vi "GEMM(LabVIEW).vi"() -> ()   [LabVIEW 2020]
uses:
  4e24d26d-fcbb-44a5-9aa8-75639d06e416.vi
  <vilib>/Analysis/baseanly.llb/Real A x B.vi
  2ed5783d-9886-4979-abaf-b24675aa47c9.vi
  <vilib>/Analysis/baseanly.llb/Mean (DBL).vi
  <vilib>/Utility/High Resolution Relative Seconds.vi
  <vilib>/Utility/file.llb/Write Delimited Spreadsheet (string).vi
  <vilib>/Analysis/NI_AALBase.lvlib
panel:
  in  "Benchmark Params":cluster{"Size":i32, "Iteration":i32}[](array[cluster])=[{"Size"=64, "Iteration"=20}, {"Size"=128, "Iteration"=20}, {"Size"=256, "Iteration"=20}, {"Size"=512, "Iteration"=20}, {"Size"=1024, "Iteration"=20}, {"Size"=2048, "Iteration"=20}, {"Size"=4096, "Iteration"=20}, {"Size"=8192, "Iteration"=3}]
  out "Results(ms)":dbl[](array[numeric])=[0.01173999989987351, 0.11100666645991926, 0.5743133331028124, 4.497079999176397, 36.276073333040884, 300.8564533326232, 2447.210946666261, 19172.94122000094] format="%.6f"
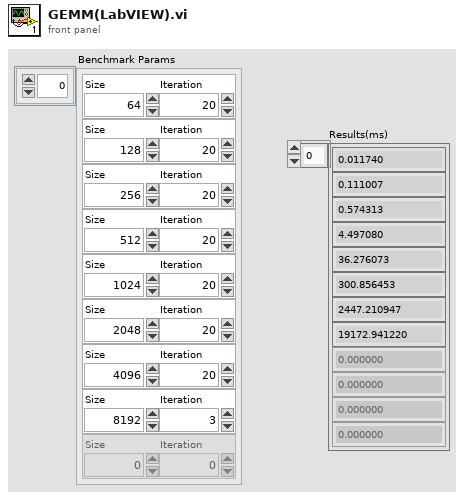
[diagram p1: front panel]
types:
  T1 = typedef "NI_Matrix.lvlib/RealMatrix.ctl" = dbl[][]
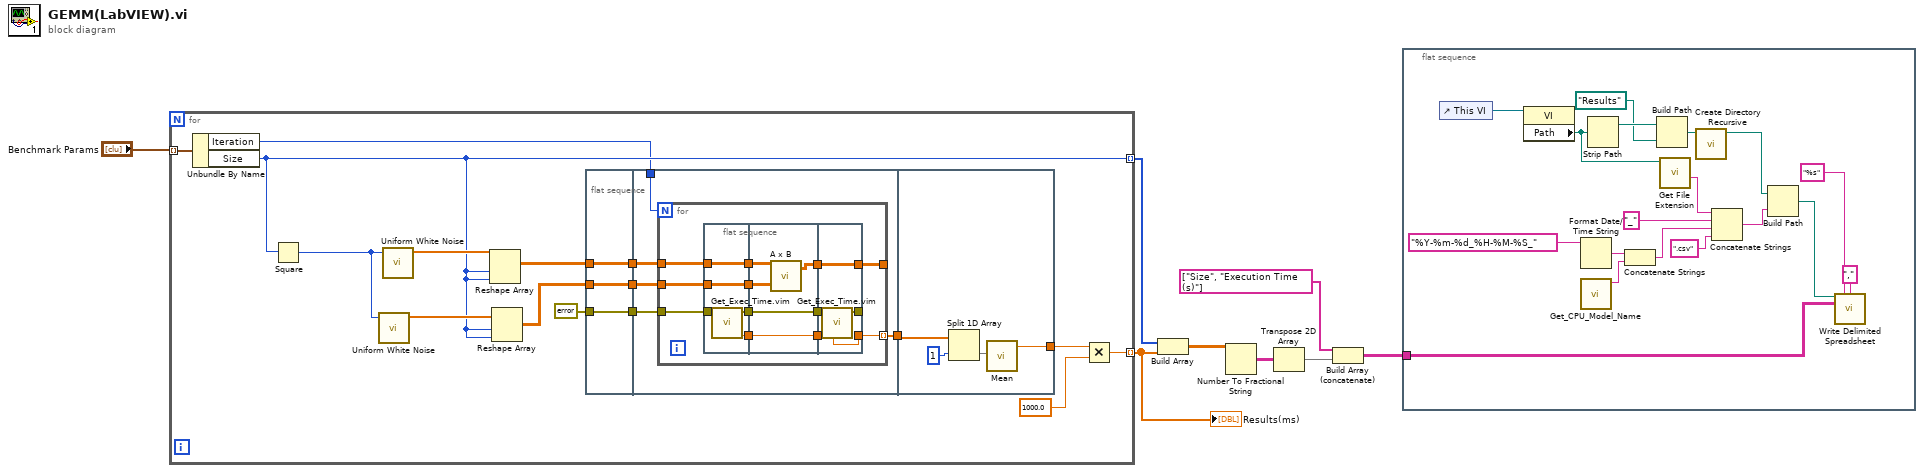
[diagram p0: block diagram]
diagram:
  n1 = for {
    tunnel: "Benchmark Params" -> [w24] mode=indexing
    tunnel: [w12] -> w8 mode=indexing
    tunnel: [w21] -> w4 mode=indexing
    n2 = Unbundle By Name(w24) -> ("Iteration"=w10:i32, "Size"=w21:i32)
    n3 = Square(x=w21) -> (x^2=w9:i32)
    n4 = call <vilib>:"Uniform White Noise.vi"("samples"=w9) -> ("uniform white noise"=w22:dbl[])  [unwired: 9 in, 1 out]
    n5 = call <vilib>:"Uniform White Noise.vi"("samples"=w9) -> ("uniform white noise"=w23:dbl[])  [unwired: 9 in, 1 out]
    n6 = Reshape Array(w23, w21, w21) -> (w17:dbl[][])
    n7 = Reshape Array(w22, w21, w21) -> (w16:dbl[][])
    n8 = flat-sequence {
      tunnel: errorcluster {"status"=FALSE, "code"=0, "source"=""} ("error out") -> [w26]
      tunnel: w17 -> [w27]
      tunnel: [w27] -> w20
      tunnel: [w26] -> w19
      tunnel: w16 -> [w25]
      tunnel: [w25] -> w15
      tunnel: w20 -> [w32]
      tunnel: w19 -> [w31]
      tunnel: [w30] -> w18
      tunnel: w15 -> [w29]
      tunnel: w10 -> [w28]
      tunnel: [w60] -> w13
      tunnel: w18 -> [w63]
      frame #0 {
      }
      frame #1 {
        n9 = for {
          N: w28 -> [_]
          tunnel: w32 -> [w44]
          tunnel: w31 -> [w42]
          tunnel: [w43] -> _
          tunnel: [w35] -> w30 mode=indexing
          tunnel: w29 -> [w34]
          n10 = flat-sequence {
            tunnel: w42 -> [w48]
            tunnel: w44 -> [w49]
            tunnel: [w49] -> w41
            tunnel: [w47] -> w40
            tunnel: [w46] -> w36
            tunnel: w34 -> [w45]
            tunnel: [w45] -> w33
            tunnel: w41 -> [w54]
            tunnel: w40 -> [w52]
            tunnel: [w53] -> w39
            tunnel: [w52] -> w38
            tunnel: [w51] -> w37
            tunnel: w36 -> [w51]
            tunnel: w33 -> [w50]
            tunnel: [w57] -> _
            tunnel: [w59] -> w43
            tunnel: w39 -> [w59]
            tunnel: w38 -> [w58]
            tunnel: w37 -> [w56]
            tunnel: [w55] -> w35
            frame #0 {
              n11 = call "Get_Exec_Time.vim"("error in (no error)"=w48) -> ("T(n)"=w46:dbl, "error out"=w47:errorcluster)  [unwired: 6 in, 1 out]
            }
            frame #1 {
              n12 = call-poly <vilib>:"A x B.vi"("B"=w50, "A"=w54) -> ("A x B"=w53:T1)  [unwired: 1 out]
            }
            frame #2 {
              n13 = call "Get_Exec_Time.vim"("T(n-1)"=w56, "error in (no error)"=w58) -> ("error out"=w57:errorcluster, "dT"=w55:dbl)  [unwired: 5 in, 1 out]
            }
          }
        }
      }
      frame #2 {
        n14 = Split 1D Array(array=w63, index=1) -> (second subarray=w61:dbl[])  [unwired: 1 out]
        n15 = call-poly <vilib>:"Mean.vi"("X"=w61) -> ("mean"=w60:dbl)  [unwired: 1 out]
      }
    }
    n16 = Multiply(x=w13, y=1000.0) -> (x*y=w12:dbl)
  }
  "Results(ms)" <- w8
  n17 = Build Array(w4, w8) -> (w7:dbl[][])
  n18 = Number To Fractional String(number=w7) -> (F-format string=w6:string[][])  [unwired: 3 in]
  n19 = Transpose 2D Array(2D array=w6) -> (transposed array=w3:string[][])
  n20 = Build Array (concatenate)(string[] ["Size", "Execution Time (s)"] ("element"), w3) -> (w1:string[][])
  n21 = flat-sequence {
    tunnel: w1 -> [w81]
    frame #0 {
      n22 = control-ref of="This VI"() -> (w75:refnum<vi>)
      n23 = property class="VI"(reference=w75) -> ("Path"=w70:path)  [unwired: 1 in, 2 out]
      n24 = Format Date/Time String(time format string (%c)="%Y-%m-%d_%H-%M-%S_") -> (date/time string=w66:string)  [unwired: 2 in]
      n25 = call "Get_CPU_Model_Name.vi"() -> ("CPU Model"=w65:string)  [unwired: 11 in]
      n26 = Strip Path(path=w70) -> (stripped path=w74:path)  [unwired: 1 out]
      n27 = Concatenate Strings(w66, w65) -> (w64:string)
      n28 = Build Path(base path=w74, name or relative path=path "Results") -> (appended path=w73:path)
      n29 = call <vilib>:"Get File Extension.vi"("file"=w70) -> ("filename without extension"=w69:string)  [unwired: 6 in, 4 out]
      n30 = call <vilib>:"Create Directory Recursive.vi"("directory"=w73) -> ("directory copy"=w71:path)  [unwired: 4 in, 2 out]
      n31 = Concatenate Strings(w69, "_" ("string"), w64, ".csv" ("string")) -> (w79:string)
      n32 = Build Path(base path=w71, name or relative path=w79) -> (appended path=w80:path)
      n33 = call-poly <vilib>:"Write Delimited Spreadsheet.vi"("file path (dialog if empty)"=w80, "format (%s)"="%s", "2D data"=w81, "delimiter (\\t)"="," ("delimiter (\\t)")) -> ()  [unwired: 10 in, 2 out]
    }
  }
